vi "Parse Limit Switch Position.vi"(11 "QS Response":string) -> (2 "At Switch?":bool, 3 "motor":i32)   [LabVIEW 2024, in "FW Arduino Control.lvclass"]
uses:
  FW Arduino Control.lvclass
  <vilib>/regexp/Match Regular Expression.xnode
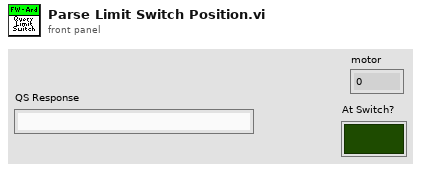
[diagram p1: front panel]
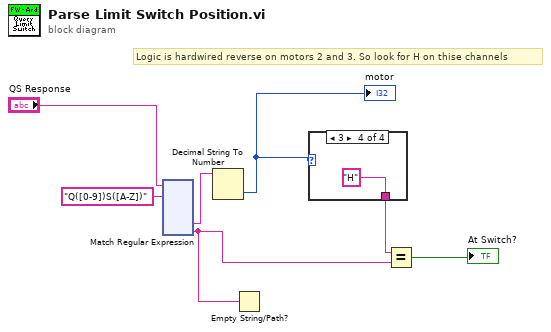
[diagram p0: block diagram]
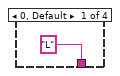
[diagram p2: hidden frame]
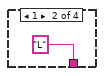
[diagram p3: hidden frame]
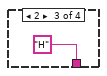
[diagram p4: hidden frame]
diagram:
  # "Logic is hardwired reverse on motors 2 and 3. So look for H on thise channels"
  n1 = xnode "Match Regular Expression"("input string"="QS Response", "regular expression"="Q([0-9])S([A-Z])") -> ("submatch 1"=w5:string, "submatch 2"=w3:string)  [unwired: 4 in, 5 out]
  n2 = Decimal String To Number(string=w5) -> (number=w2:i32)  [unwired: 2 in, 1 out]
  "motor" <- w2
  n3 = Empty String/Path?(string/path=w3) -> ()  [unwired: 1 out]
  n4 = case shown="3" w2 {
    tunnel: ["L" ("y") "L" ("y") "H" ("y") "H" ("y")] -> w1
    frame 0, Default {
    }
    frame 1 {
    }
    frame 2 {
    }
    frame 3 {
    }
  }
  n5 = Equal?(x=w1, y=w3) -> (x = y?=→"At Switch?":bool)
